vi "ScanSpectrum.vi"(8 "error in":errorcluster, 11 "StellarNetSpecAcquisition in":refnum<class "StellarNetSpecAcquisition.lvclass">) -> (0 "error out":errorcluster, 3 "StellarNetSpecAcquisition out":refnum<class "StellarNetSpecAcquisition.lvclass">)   [LabVIEW 2020, in "StellarNetSpecAcquisition.lvclass"]
doc: "Phisically read the data from the device assigned to the current session"
uses:
  StellarNetSpecAcquisition.lvclass
  StellarNetSpecAcquisition.lvclass/StellarNetSpecAcquisition.ctl
  StellarNetSpectrometerClass/StellarNetSpectrometer.lvclass
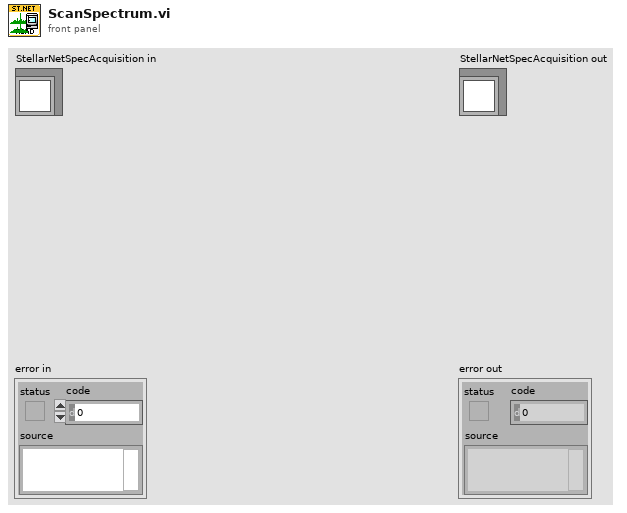
[diagram p1: front panel]
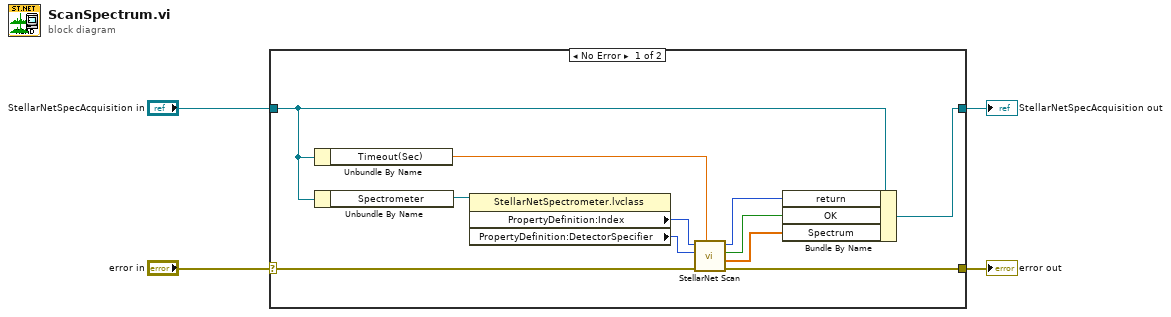
[diagram p0: block diagram]
diagram:
  n1 = case shown="No Error" "error in" {
    selector: "error in" -> [w15 w17]
    tunnel: [w14 w17] -> w3
    tunnel: [w5 w16] -> w1
    tunnel: "StellarNetSpecAcquisition in" -> [w9 w16]
    frame No Error {
      n2 = Unbundle By Name(w9) -> ("Timeout(Sec)"=w10:dbl)
      n3 = Unbundle By Name(w9) -> ("Spectrometer"=w13:refnum<class "StellarNetSpectrometer.lvclass">)
      n4 = property class="StellarNetSpectrometer.lvclass"(reference=w13) -> ("PropertyDefinition:Index"=w12:u32, "PropertyDefinition:DetectorSpecifier"=w11:u16)  [unwired: 1 in, 2 out]
      n5 = call "StellarNet Scan.vi"("Timeout(Sec)"=w10, "error in"=w15, "DetectorSpecifier"=w11, "Index"=w12) -> ("error out"=w14:errorcluster, "Spectrum"=w6:sgl[], "OK"=w7:bool, "return"=w8:i32)  [unwired: 4 in]
      n6 = Bundle By Name(cluster=w9, "return"=w8, "OK"=w7, "Spectrum"=w6) -> (w5:refnum<class "StellarNetSpecAcquisition.lvclass">)
    }
    frame Error {
    }
  }
  "error out" <- w3
  "StellarNetSpecAcquisition out" <- w1
